vi "Grab images from pco.edge or pco.pixelfly USB.vi"() -> ()   [LabVIEW 2012]
doc: "A short program to demonstrate the fundamentals of control and image acquision with the pco.camera series. The program records a sequence of images, with \"live\" updating, until the \"StopRecording\" button is pressed. Use ctrl-H for more help on the individual controls and indicators.\n\nCopyright 2004, 2010 The Cooke Corporation."
panel:
  out "bClose":bool
  in  "Quit":bool
  out "BufNr1":i16
  out "BufNr0":i16
  in  "bUseBuffer1":bool
  in  "bUseBuffer0":bool
  in  "ROIX1":u16=1 min=1
  in  "ROIY1":u16=1 min=1
  in  "ROIY0":u16=1 min=1
  in  "ROIX0":u16=1 min=1
  out "Bits/pixel":u16
  in  "Record":bool
  in  "DelayTimeBase":u16(ring)=2 items=["nanoseconds", "microseconds", "milliseconds"]
  in  "ExposureTimeBase":u16(ring)=2 items=["nanoseconds", "microseconds", "milliseconds"]
  in  "Exposure":u32=10
  in  "Delay":u32
  in  "Rate":i32(ring) items=["12000000", "25000000", "0", "0"]
  out "Image":u16[][](graph)
  in  "TriggerMode":u16(ring) items=["Auto", "Software", "External sequence start ", "External exposure control"]
  # "A short program to demonstrate the fundamentals of control and image acquision with the pco.camera series. The program records a sequence of images, with \"live\" updating, until the \"StopRecording\" button is pressed.  Use ctrl-H for more help on the individual controls and indicators."
  # "pco.labview"
  # "1) Setup camera:"
  # "2) Record  images:"
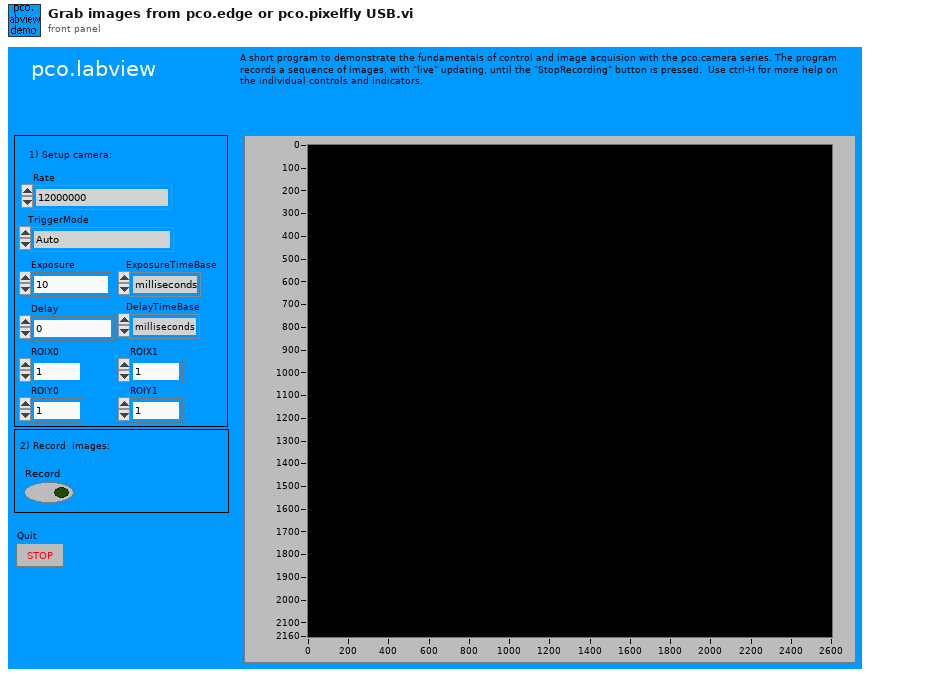
[diagram p1: front panel]
types:
  T1 = cluster{"Size":u16, "CamType":u16, "CamSubType":u16, "SerialNumber":u32, "HWVersion":u32, "FWVersion":u32, "InterfaceType":u16, "HardwareVersion":cluster{"BoardNum":u16, "HWVersions":cluster{"BoardName":string, "BatchNumber":u16, "MinorRevision":u8, "MajorRevision":u8, "Variant":u16}[]}, "FirmwareVersion":cluster{"DeviceNum":u16, "FWVersions":cluster{"DeviceName":string, "MinorRevision":u8, "MajorRevision":u8, "Variant":u16}[]}}
  T2 = cluster{"Size":u16, "SensorTypeDESC":u16, "SensorSubtypeDESC":u16, "MaxHorizontalResStdDESC":u16, "MaxVerticalResStdDESC":u16, "MaxHorizontalResExtDESC":u16, "MaxVerticalResExtDESC":u16, "DynResDESC":u16, "MaxBinHorzDESC":u16, "BinHorzStepDESC":bool, "MaxBinVertDESC":u16, "BinVertStepDESC":bool, "ROIHorzStepDESC":u16, "ROIVertStepDESC":u16, "NumADCDESC":u16, "IRDESC":bool, "MinDelayDESC":u32, "MaxDelayDESC":u32, "MinDelayStepDESC":u32, "MinExpoDESC":u32, "MaxExpoDESC":u32, "MinExpoStepDESC":u32, "MinDelayIRDESC":u32, "MaxDelayIRDESC":u32, "MinExpoIRDESC":u32, "MaxExpoIRDESC":u32, "TimeTableDESC":bool, "DoubleImageDESC":bool, "MinCoolSetDESC":i16, "MaxCoolSetDESC":i16, "MDefaultCoolSetDESC":i16, "PowerDownModeDESC":bool, "OffsetRegDESC":bool, "ColorPattern":cluster{"UpperLeftColor":u8, "UpperRightColor":u8, "LowerLeftColor":u8, "LowerRightColor":u8}, "PatternTypeDESC":bool, "PixelRates":u32[], "CoversionFactors":u16[], "Reserved":u32[], "NoiseFilterCapable":bool, "HotPixelCapable":bool, "HotPixelWithNoiseFilter":bool, "ASCIITimeCapable":bool, "Extended Description":bool, "Get Extended":bool, "Reserved Flag 1":bool, "Reserved Flag 2":bool}
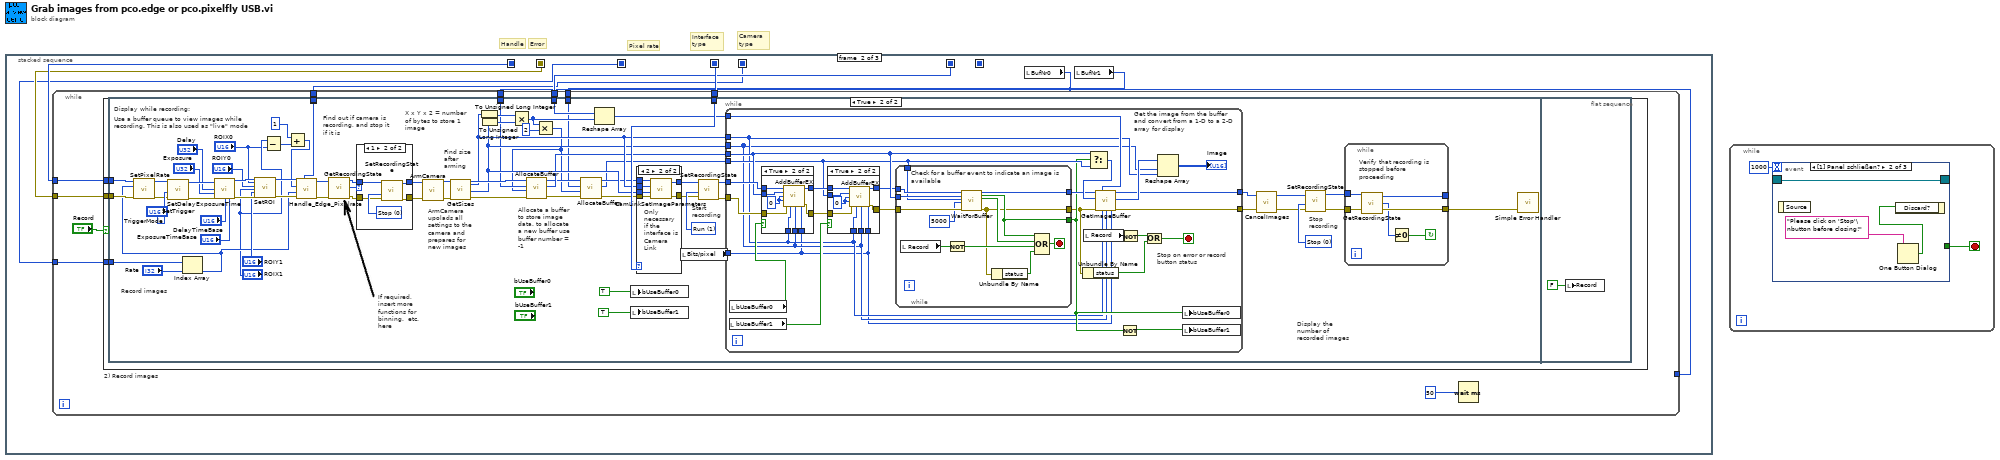
[diagram p0: block diagram]
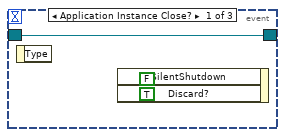
[diagram p2: hidden frame]
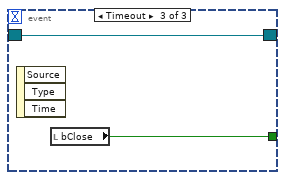
[diagram p3: hidden frame]
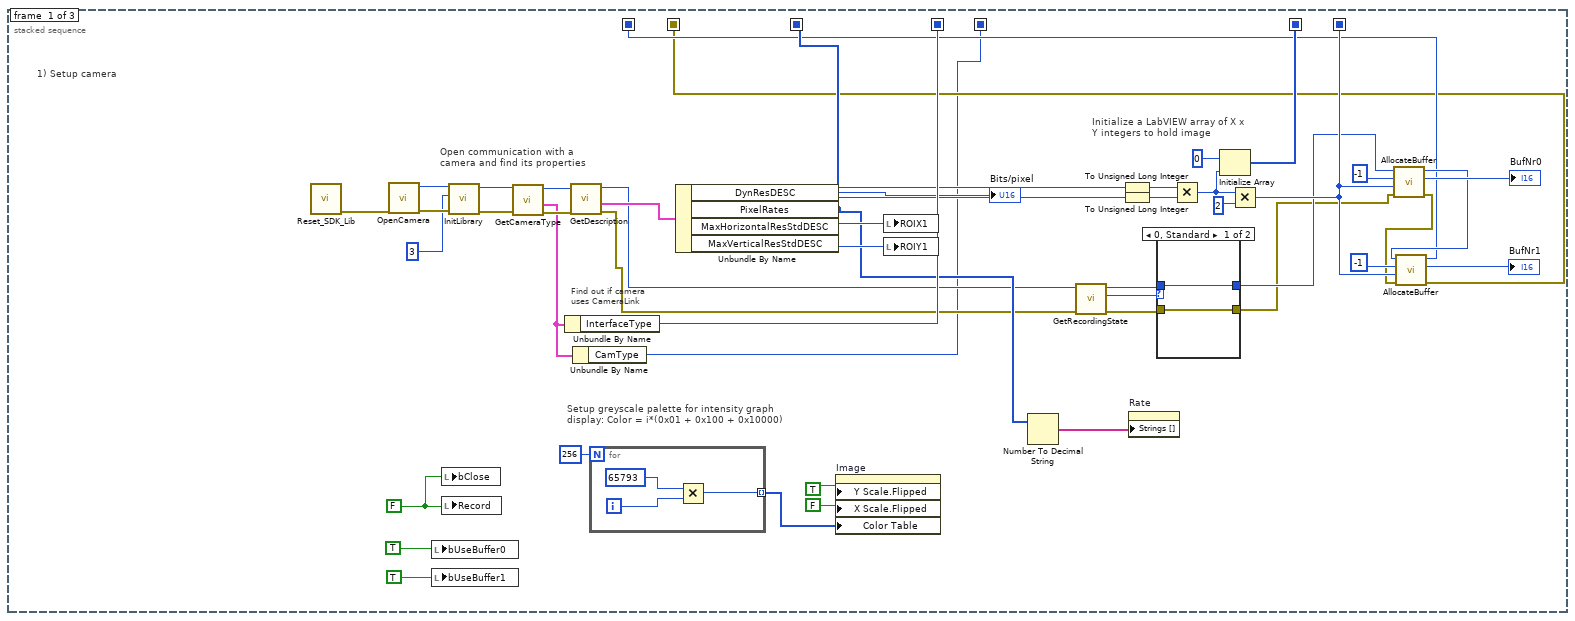
[diagram p4: hidden frame]
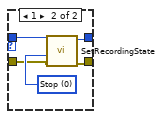
[diagram p5: hidden frame]
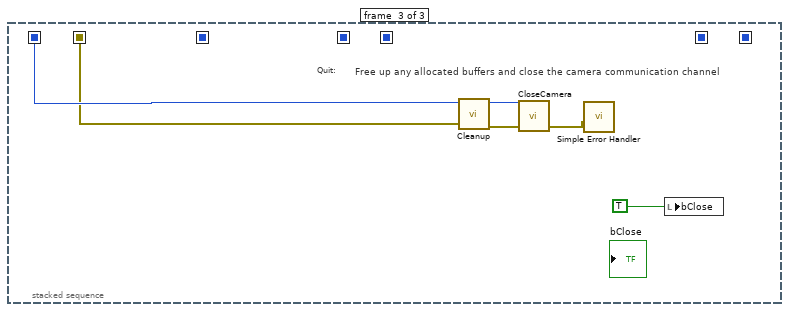
[diagram p11: hidden frame]
diagram:
  # "Camera type"
  # "Interface type"
  # "Error"
  # "Handle"
  # "Pixel rate"
  n1 = stacked-sequence {
    seq-local: [w40 _ _] -> [_ w61 _]
    seq-local: [w28 _ _] -> [_ _ _]
    seq-local: [w7 _ _] -> [_ w64 w240]
    seq-local: [w6 _ _] -> [_ w63 w239]
    seq-local: [w35 _ _] -> [_ w62 _]
    seq-local: [w20 _ _] -> [_ w58 _]
    seq-local: [w1 _ _] -> [_ w57 _]
    frame #0 {
      w22 = FALSE ("stop")
      # "1) Setup camera"
      # "Find out if camera uses CameraLink"
      # "Setup greyscale palette for intensity graph display: Color = i*(0x01 + 0x100 + 0x10000)"
      # "Initialize a LabVIEW array of X x Y integers to hold image"
      # "Open communication with a camera and find its properties"
      n2 = call "Reset_SDK_Lib.vi"() -> ("ErrorOut"=w3:errorcluster)  [unwired: 11 in]
      n3 = call "OpenCamera.vi"("ErrorIn"=w3) -> ("ErrorOut"=w18:errorcluster, "Handle out"=w19:u64)  [unwired: 3 in, 2 out]
      n4 = local write "bUseBuffer0"(TRUE) -> ()
      n5 = local write "bUseBuffer1"(TRUE) -> ()
      n6 = local write "bClose"(w22) -> ()
      n7 = local write "Record"(w22) -> ()
      n8 = call "InitLibrary.vi"("error in (no error)"=w18, "InterfaceType"=u32 3, "ph"=w19) -> ("error out"=w17:errorcluster, "hout"=w16:u64)  [unwired: 7 in]
      n9 = call "GetCameraType.vi"("ph"=w16, "error in (no error)"=w17) -> ("hout"=w37:u64, "CameraType"=w2:T1, "error out"=w36:errorcluster)  [unwired: 1 in, 1 out]
      n10 = Unbundle By Name(w2) -> ("InterfaceType"=w35:u16)
      n11 = call "GetDescription.vi"("ErrorIn"=w36, "ph"=w37) -> ("ErrorOut"=w13:errorcluster, "Description"=w39:T2, "hout"=w12:u64)  [unwired: 2 in, 1 out]
      n12 = Unbundle By Name(w2) -> ("CamType"=w1:u16)
      n13 = for {
        N: 256 -> [_]
        tunnel: [w54] -> w43 mode=indexing
        i -> [w55]
        n14 = Multiply(x=65793, y=w55) -> (x*y=w54:i32)
      }
      n15 = Unbundle By Name(w39) -> ("DynResDESC"=→"Bits/pixel":u16, "PixelRates"=w20:u32[], "MaxHorizontalResStdDESC"=w33:u16, "MaxVerticalResStdDESC"=w32:u16)
      n16 = property on="Image" class="IntGraph (strikt)"("Y Scale.Flipped"=TRUE, "X Scale.Flipped"=FALSE, "Color Table"=w43) -> ()  [unwired: 2 in, 2 out]
      n17 = local write "ROIX1"(w33) -> ()
      n18 = local write "ROIY1"(w32) -> ()
      n19 = Number To Decimal String(number=w20) -> (decimal integer string=w21:string[])  [unwired: 1 in]
      n20 = call "GetRecordingState.vi"("ErrorIn"=w13, "ph"=w12) -> ("ErrorOut"=w10:errorcluster, "Error"=w4:i32, "hout"=w11:u64)  [unwired: 2 in, 1 out]
      n21 = To Unsigned Long Integer(number=w33) -> (unsigned 32bit integer=w30:u32)
      n22 = To Unsigned Long Integer(number=w32) -> (unsigned 32bit integer=w29:u32)
      n23 = property on="Rate" class="Ring (strikt)"("Strings []"=w21) -> ()  [unwired: 2 in, 2 out]
      n24 = case shown="0, Standard" w4 {
        tunnel: w11 -> [w48 w52]
        tunnel: w10 -> [w47 w51]
        tunnel: [w48 w50] -> w9
        tunnel: [w47 w49] -> w5
        frame 0, Default {
        }
        frame 1 {
          w53 = u16 0 items=["Stop", "Run"] ("RecordingState")
          n25 = call "SetRecordingState.vi"("ErrorIn"=w51, "RecordingState"=w53, "ph"=w52) -> ("ErrorOut"=w49:errorcluster, "hout"=w50:u64)  [unwired: 2 in, 1 out]
        }
      }
      n26 = Multiply(x=w30, y=w29) -> (x*y=w41:u32)
      n27 = Initialize Array(u16 0 ("Element Data"), w41) -> (w40:u16[])
      n28 = Multiply(x=w41, y=u32 2) -> (x*y=w28:u32)
      n29 = call "AllocateBuffer.vi"("error in (no error)"=w5, "Size"=w28, "BufNr"=i16 -1, "ph"=w9) -> ("error out"=w14:errorcluster, "BufNrOut"=→"BufNr0":i16, "hout"=w8:u64)  [unwired: 2 in, 3 out]
      n30 = call "AllocateBuffer.vi"("error in (no error)"=w14, "Size"=w28, "BufNr"=i16 -1, "ph"=w8) -> ("error out"=w6:errorcluster, "BufNrOut"=→"BufNr1":i16, "hout"=w7:u64)  [unwired: 2 in, 3 out]
    }
    frame #1 {
      n31 = local read "BufNr0"() -> (w60:i16)
      n32 = local read "BufNr1"() -> (w59:i16)
      n33 = while {
        tunnel: w60 -> [_]
        tunnel: w60 -> [w70]
        tunnel: w61 -> [w72]
        tunnel: w62 -> [w73]
        tunnel: w63 -> [w71]
        tunnel: w64 -> [w68]
        tunnel: w59 -> [w69]
        tunnel: w58 -> [w66]
        tunnel: w57 -> [w65]
        stop <- "Quit" stop-if-true
        n34 = case "2) Record images" shown="True" "Record" {
          tunnel: w68 -> [_ w83]
          tunnel: w71 -> [_ w82]
          tunnel: w73 -> [_ w81]
          tunnel: w72 -> [_ w80]
          tunnel: w70 -> [_ w79]
          tunnel: w69 -> [_ w78]
          tunnel: w66 -> [_ w77]
          tunnel: w65 -> [_ w76]
          frame False {
          }
          frame True {
            n35 = flat-sequence {
              tunnel: w83 -> [w132]
              tunnel: w82 -> [w131]
              tunnel: w81 -> [w129]
              tunnel: w80 -> [w127]
              tunnel: w79 -> [w114]
              tunnel: w78 -> [w108]
              tunnel: w77 -> [w95]
              tunnel: w76 -> [w84]
              frame #0 {
                w151 = u16 1 items=["Stop", "Run"] ("RecordingState")
                w154 = u16 0 items=["Stop", "Run"] ("RecordingState")
                # "Display the number of recorded images"
                # "Record images"
                # "Start recording"
                # "Allocate a buffer to store image data. to allocate a new buffer use buffer number = -1"
                # "Find size after arming"
                # "ArmCamera upolads all settings to the camera and prepares for new images"
                # "Find out if camera is recording, and stop it if it is"
                # "If required, insert more functions for binning.  etc. here"
                # "X x Y x 2 = number of bytes to store 1 image"
                # "Stop recording"
                # "Use a buffer queue to view images while recording. This is also used as \"live\" mode"
                # "Display while recording:"
                n36 = Index Array(array=w95, index="Rate") -> (element=w90:u32)
                n37 = call "SetPixelRate.vi"("error in (no error)"=w131, "PixelRate"=w90, "ph"=w132) -> ("error out"=w97:errorcluster, "hout"=w98:u64)  [unwired: 2 in, 1 out]
                n38 = call "SetTrigger.vi"("error in (no error)"=w97, "TriggerMode"="TriggerMode", "ph"=w98) -> ("error out"=w139:errorcluster, "hout"=w140:u64)  [unwired: 2 in, 1 out]
                n39 = call "SetDelayExposureTime.vi"("ph"=w140, "Delay"="Delay", "Exposure"="Exposure", "error in (no error)"=w139, "DelayTimeBase"="DelayTimeBase", "ExposureTimeBase"="ExposureTimeBase") -> ("hout"=w118:u64, "error out"=w117:errorcluster)  [unwired: 7 in, 1 out]
                n40 = call "SetROI.vi"("ph"=w118, "ROIX0"="ROIX0", "ROIY0"="ROIY0", "ROIX1"="ROIX1", "ROIY1"="ROIY1", "error in (no error)"=w117) -> ("hout"=w91:u64, "error out"=w92:errorcluster)  [unwired: 12 in]
                n41 = Subtract(x="ROIX1", y="ROIX0") -> (x-y=w87:u16)
                n42 = Add(x=1, y=w87) -> (x+y=w85:i32)
                n43 = call "Handle_Edge_Pixelrate.vi"("Cameratype"=w84, "error in (no error)"=w92, "PixelRate"=w90, "X-Resolution"=w85, "ph"=w91) -> ("error out"=w93:errorcluster, "hout"=w94:u64)  [unwired: 5 in]
                n44 = call "GetRecordingState.vi"("ErrorIn"=w93, "ph"=w94) -> ("ErrorOut"=w148:errorcluster, "RecordingState"=w150:u16, "hout"=w149:u64)  [unwired: 2 in, 1 out]
                n45 = case shown="1" w150 {
                  tunnel: w149 -> [w232 w236]
                  tunnel: w148 -> [w231 w235]
                  tunnel: [w232 w234] -> w147
                  tunnel: [w231 w233] -> w146
                  frame 0, Default {
                  }
                  frame 1 {
                    w237 = u16 0 items=["Stop", "Run"] ("RecordingState")
                    n46 = call "SetRecordingState.vi"("ErrorIn"=w235, "RecordingState"=w237, "ph"=w236) -> ("ErrorOut"=w233:errorcluster, "hout"=w234:u64)  [unwired: 2 in, 1 out]
                  }
                }
                n47 = call "ArmCamera.vi"("error in (no error)"=w146, "ph"=w147) -> ("error out"=w144:errorcluster, "hout"=w145:u64)  [unwired: 1 in, 1 out]
                n48 = call "GetSizes.vi"("ph"=w145, "ErrorIn"=w144) -> ("hout"=w141:u64, "XResAct"=w125:u16, "YResAct"=w124:u16, "ErrorOut"=w143:errorcluster)  [unwired: 11 in, 3 out]
                n49 = To Unsigned Long Integer(number=w125) -> (unsigned 32bit integer=w119:u32)
                n50 = To Unsigned Long Integer(number=w124) -> (unsigned 32bit integer=w120:u32)
                n51 = Multiply(x=w119, y=w120) -> (x*y=w121:u32)
                n52 = Multiply(x=w121, y=u32 2) -> (x*y=w109:u32)
                n53 = call "AllocateBuffer.vi"("error in (no error)"=w143, "Size"=w109, "BufNr"=w114, "ph"=w141) -> ("error out"=w113:errorcluster, "BufNrOut"=w122:i16, "hout"=w111:u64)  [unwired: 2 in, 3 out]
                n54 = call "AllocateBuffer.vi"("error in (no error)"=w113, "Size"=w109, "BufNr"=w108, "ph"=w111) -> ("error out"=w112:errorcluster, "BufNrOut"=w107:i16, "hout"=w110:u64)  [unwired: 2 in, 3 out]
                n55 = Reshape Array(w127, w121) -> (w126:u16[])
                n56 = local write "bUseBuffer0"(TRUE) -> ()
                n57 = local write "bUseBuffer1"(TRUE) -> ()
                n58 = case shown="2" w129 {
                  tunnel: w112 -> [w223 w230]
                  tunnel: [w223 w229] -> w134
                  tunnel: w110 -> [w224 w228]
                  tunnel: [w224 w227] -> w133
                  tunnel: w124 -> [_ w226]
                  tunnel: w125 -> [_ w225]
                  frame 0, Default {
                  }
                  frame 2 {
                    # "Only necessary if the interface is Camera Link"
                    n59 = call "CamLinkSetImageParameters.vi"("error in (no error)"=w230, "YRes"=w226, "XRes"=w225, "ph"=w228) -> ("error out"=w229:errorcluster, "hout"=w227:u64)  [unwired: 1 out]
                  }
                }
                n60 = local read "Bits/pixel"() -> (w102:u16)
                n61 = call "SetRecordingState.vi"("ErrorIn"=w134, "RecordingState"=w151, "ph"=w133) -> ("ErrorOut"=w130:errorcluster, "hout"=w128:u64)  [unwired: 2 in, 1 out]
                n62 = while {
                  tunnel: w122 -> [w167]
                  tunnel: w126 -> [w177]
                  tunnel: w128 -> [w176]
                  tunnel: w124 -> [w156]
                  tunnel: w125 -> [w157]
                  tunnel: w130 -> [w174]
                  tunnel: [w179] -> w101
                  tunnel: [w180] -> w100
                  tunnel: w107 -> [w166]
                  tunnel: w102 -> [w155]
                  stop <- w158 stop-if-true
                  # "Stop on error or record button status"
                  # "Get the image from the buffer and convert from a 1-D to a 2-D array for display"
                  n63 = local read "bUseBuffer1"() -> (w171:bool)
                  n64 = local read "bUseBuffer0"() -> (w172:bool)
                  n65 = case shown="True" w172 {
                    tunnel: [w183 w192] -> w173
                    tunnel: [w182 w191] -> w175
                    tunnel: w167 -> [_ w190]
                    tunnel: w176 -> [w182 w189]
                    tunnel: w155 -> [_ w187]
                    tunnel: w157 -> [_ w186]
                    tunnel: w156 -> [_ w185]
                    tunnel: w174 -> [w183 w184]
                    frame False {
                    }
                    frame True {
                      w188 = i16 0
                      n66 = call "AddBufferEX.vi"("ph"=w189, "BuffNr"=w190, "1stImage"=w188, "LastImage"=w188, "error in (no error)"=w184, "XRes"=w186, "YRes"=w185, "BitPerPixel"=w187) -> ("hout"=w191:u64, "error out"=w192:errorcluster)  [unwired: 5 in, 1 out]
                    }
                  }
                  n67 = case shown="True" w171 {
                    tunnel: [w193 w203] -> w164
                    tunnel: [w194 w202] -> w165
                    tunnel: w166 -> [_ w201]
                    tunnel: w175 -> [w194 w200]
                    tunnel: w155 -> [_ w198]
                    tunnel: w157 -> [_ w197]
                    tunnel: w156 -> [_ w196]
                    tunnel: w173 -> [w193 w195]
                    frame False {
                    }
                    frame True {
                      w199 = i16 0
                      n68 = call "AddBufferEX.vi"("ph"=w200, "BuffNr"=w201, "1stImage"=w199, "LastImage"=w199, "error in (no error)"=w195, "XRes"=w197, "YRes"=w196, "BitPerPixel"=w198) -> ("hout"=w202:u64, "error out"=w203:errorcluster)  [unwired: 5 in, 1 out]
                    }
                  }
                  n69 = while {
                    tunnel: w167 -> [w211]
                    tunnel: w166 -> [w210]
                    tunnel: w165 -> [w213]
                    tunnel: w164 -> [w212]
                    tunnel: [w209] -> w163
                    tunnel: [w205] -> w161
                    tunnel: [w208] -> w162
                    stop <- w214 stop-if-true
                    # "Check for a buffer event to indicate an image is available"
                    n70 = local read "Record"() -> (w216:bool)
                    n71 = Not(x=w216) -> (.not. x?=w215:bool)
                    n72 = call "WaitForBuffer.vi"("ph"=w213, "sBufNr"=w211, "sBufNr 2"=w210, "timeout"=5000, "error in (no error)"=w212) -> ("hout"=w209:u64, "Buffer_Ready"=w208:bool, "Buffer_Ready 2"=w207:bool, "error out"=w205:errorcluster)  [unwired: 10 in, 1 out]
                    n73 = Unbundle By Name(w205) -> ("status"=w204:bool)
                    n74 = Compound Arithmetic op=OR(w208, w207, w215, w204) -> (w214:bool)
                  }
                  n75 = Unbundle By Name(w161) -> ("status"=w159:bool)
                  n76 = local read "Record"() -> (w178:bool)
                  n77 = Select(t=w167, s=w162, f=w166) -> (s? t:f=w170:i16)
                  n78 = call "GetImageBuffer.vi"("ph"=w163, "BuffIn"=w177, "BuffNr"=w170, "error in (no error)"=w161, "xRes"=w157, "yRes"=w156, "Bitresolution"=w155) -> ("hout"=w179:u64, "BuffOut"=w181:u16[], "error out"=w180:errorcluster)  [unwired: 5 in, 1 out]
                  n79 = Not(x=w162) -> (.not. x?=w169:bool)
                  n80 = Not(x=w178) -> (.not. x?=w160:bool)
                  n81 = Or(x=w160, y=w159) -> (x .or. y?=w158:bool)
                  n82 = Reshape Array(w181, w156, w157) -> (→"Image":u16[][])
                  n83 = local write "bUseBuffer0"(w162) -> ()
                  n84 = local write "bUseBuffer1"(w169) -> ()
                }
                n85 = call "CancelImages.vi"("error in (no error)"=w100, "ph"=w101) -> ("error out"=w104:errorcluster, "hout"=w103:u64)  [unwired: 1 in, 1 out]
                n86 = call "SetRecordingState.vi"("ErrorIn"=w104, "RecordingState"=w154, "ph"=w103) -> ("ErrorOut"=w152:errorcluster, "hout"=w153:u64)  [unwired: 2 in, 1 out]
                n87 = while {
                  tunnel: [w220] -> w99
                  tunnel: w152 -> [w221]
                  tunnel: w153 -> [w222]
                  tunnel: [w217] -> _
                  stop <- w218 continue-if-true
                  # "Verify that recording is stopped before proceeding"
                  n88 = call "GetRecordingState.vi"("ErrorIn"=w221, "ph"=w222) -> ("ErrorOut"=w220:errorcluster, "RecordingState"=w219:u16, "hout"=w217:u64)  [unwired: 2 in, 1 out]
                  n89 = Not Equal To 0?(x=w219) -> (x != 0?=w218:bool)
                }
                n90 = call <vilib>:"Simple Error Handler.vi"("error in (no error)"=w99) -> ()  [unwired: 4 in, 5 out]
              }
              frame #1 {
                n91 = local write "Record"(FALSE ("Record")) -> ()
              }
            }
          }
        }
        n92 = Wait (ms)(milliseconds to wait=u32 50) -> ()  [unwired: 1 out]
      }
    }
    frame #2 {
      # "Free up any allocated buffers and close the camera communication channel"
      # "Quit:"
      n93 = call "Cleanup.vi"("error in (no error)"=w239, "ph"=w240) -> ("error out"=w241:errorcluster, "hout"=w242:u64)  [unwired: 8 in]
      n94 = call "CloseCamera.vi"("ErrorIn"=w241, "Handle in"=w242) -> ("ErrorOut"=w244:errorcluster)  [unwired: 1 in, 2 out]
      n95 = call <vilib>:"Simple Error Handler.vi"("error in (no error)"=w244) -> ()  [unwired: 4 in, 5 out]
      n96 = local write "bClose"(TRUE) -> ()
    }
  }
  n97 = while {
    stop <- w245 stop-if-true
    n98 = event shown="[1] Panel schließen?" {
      selector: _ -> [w247 w252 w254]
      dyn-events: [w247 w252 w254] -> _
      timeout: 1000 -> [_ _ _]
      tunnel: [_ _ w253] -> w245
      event Application Instance Close? {
        n99 = event-data() -> ()  [unwired: 1 in, 1 out]
        n100 = event-data("SilentShutdown"=FALSE, "Discard?"=TRUE) -> ()  [unwired: 1 in, 1 out]
      }
      event Panel Close? {
        n101 = event-data() -> ()  [unwired: 1 in, 1 out]
        n102 = One Button Dialog(message="Please click on 'Stop'\nbutton before closing!") -> (true=w250:bool)  [unwired: 1 in]
        n103 = event-data("Discard?"=w250) -> ()  [unwired: 1 in, 1 out]
      }
      event Timeout {
        n104 = event-data() -> ()  [unwired: 1 in, 3 out]
        n105 = local read "bClose"() -> (w253:bool)
      }
    }
  }
